vi "Bidirectional Circular Count (SubVI).vi"(7 "Max. Count":u16, 11 "Count In":i16) -> (3 "Count Out":i16)   [LabVIEW 2015]
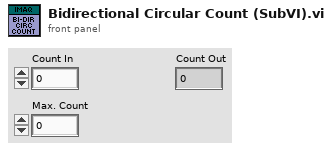
[diagram p1: front panel]
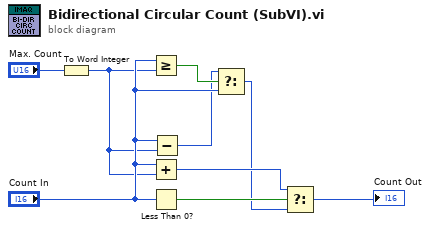
[diagram p0: block diagram]
diagram:
  n1 = To Word Integer(number="Max. Count") -> (16bit integer=w2:i16)
  n2 = Greater Or Equal?(x="Count In", y=w2) -> (x >= y?=w8:bool)
  n3 = Add(x="Count In", y=w2) -> (x+y=w6:i16)
  n4 = Less Than 0?(x="Count In") -> (x < 0?=w7:bool)
  n5 = Subtract(x="Count In", y=w2) -> (x-y=w1:i16)
  n6 = Select(t=w1, s=w8, f="Count In") -> (s? t:f=w4:i16)
  n7 = Select(t=w6, s=w7, f=w4) -> (s? t:f=→"Count Out":i16)
